vi "Execute Multiple Commands with a Single Channel with a Raspberry Pi.vi"() -> ()   [LabVIEW 2018]
doc: "Executes a multiple commands using a single channel with a Raspberry Pi as the remote SSH server. This is similar to connecting to a Raspberry Pi and executing multiple sequential commands. A more interactive experience, like a Read-Evaluate-Print-Loop (REPL), would require a while loop and some more complexity."
uses:
  Toolkit/Channel/Type Definitions/Terminals.ctl
  Toolkit/Channel/Channel.lvclass/Channel.ctl
  Toolkit/Session/Session.lvclass/Session.ctl
  Toolkit/SSH/SSH.lvclass/SSH.ctl
  Toolkit/Session/Utility/Read Shared Library.vi
  Toolkit/SSH/Utility/Read Shared Library.vi
  Toolkit/Session/Support/Create from SSH.vi
  Toolkit/Session/Support/Password Authentication.vi
  Toolkit/Channel/Support/Create from Session.vi
  Toolkit/Support/Check Status.vi
  Toolkit/Channel/Support/Destroy to Session.vi
  Toolkit/Session/Support/Destroy to SSH.vi
  Toolkit/SSH/SSH.lvclass
  Toolkit/Session/Session.lvclass
  Toolkit/Channel/Channel.lvclass
panel:
  out "Login Message":string
  out "Response 2":string
  in  "Command 2":string="echo \"Hello World from the second command!\""
  out "Response 1":string
  in  "Command 1":string="echo \"Hello World from the first command!\""
  in  "Raspberry Pi Address":string="raspberrypi.local"
  in  "Password":string
  in  "Username":string="pi"
  # "Overview: Demonstrates executing a multiple, sequential commands using a single Shell channel with a Raspberry Pi\nInstructions:\n1. Change the Raspberry Pi Address from the mDNS default to another mDNS or the IP address of the Raspberry Pi if needed.\n2. Change the username from the default Raspberry Pi user if needed.\n3. Enter the password for the Raspberry Pi user.\n4. Run this VI.\n5. Observe the login message from the Raspberry Pi.\n6. Observe \"Hello World from the first command!\" and \"Hello World from the second command!\" for Response 1 and 2, respectively.\n7. Change Command 1 and Command 2.\n8. Rerun this VI.\n9. Observe the responses for Command 1 and Command 2, respectively."
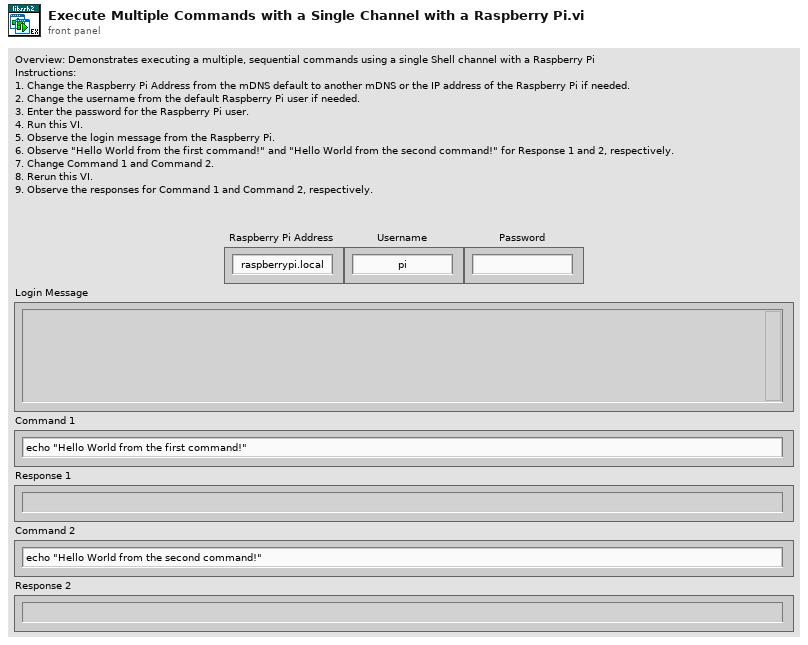
[diagram p1: front panel]
types:
  T1 = typedef "Toolkit.lvlib/Channel.lvclass/Terminals.ctl" = enum16{"ansi", "dump", "linux", "rxvt", "screen", "sun", "vt100", "vt102", "vt220", "vt52", "xterm"}
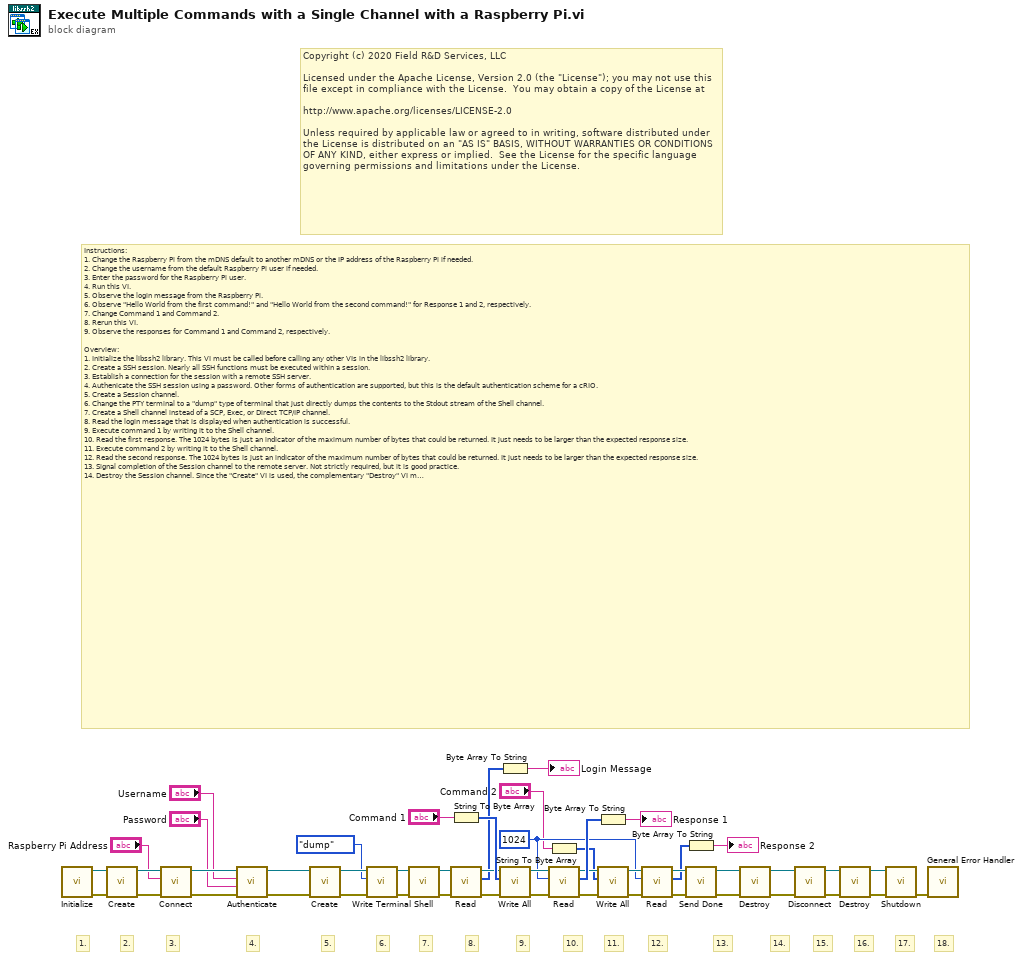
[diagram p0: block diagram]
diagram:
  w13 = u64 1024 ("Max Data Length")
  # "18."
  # "Copyright (c) 2020 Field R&D Services, LLC\n\nLicensed under the Apache License, Version 2.0 (the \"License\"); you may not use this file except in compliance with the License.  You may obtain a copy of the License at\n\nhttp://www.apache.org/licenses/LICENSE-2.0\n\nUnless required by applicable law or agreed to in writing, software distributed under the License is distributed on an \"AS IS\" BASIS, WITHOUT WARRANTIES OR CONDITIONS OF ANY KIND, either express or implied.  See the License for the specific language governing permissions and limitations under the License."
  # "17."
  # "16."
  # "15."
  # "14."
  # "13."
  # "12."
  # "11."
  # "10."
  # "9."
  # "8."
  # "7."
  # "6."
  # "5."
  # "4."
  # "3."
  # "2."
  # "1."
  # "Instructions:\n1. Change the Raspberry Pi from the mDNS default to another mDNS or the IP address of the Raspberry Pi if needed.\n2. Change the username from the default Raspberry Pi user if needed.\n3. Enter the password for the Raspberry Pi user.\n4. Run this VI.\n5. Observe the login message from the Raspberry Pi.\n6. Observe \"Hello World from the first command!\" and \"Hello World from the second command!\" for Response 1 and 2, respectively.\n7. Change Command 1 and Command 2.\n8. Rerun this VI.\n9. Observe the responses for Command 1 and Command 2, respectively.\n\nOverview:\n1. Initialize the libssh2 library. This VI must be called before calling any other VIs in the libssh2 library.\n2. Create a SSH session. Nearly all SSH functions must be executed within a session.\n3. Establish a connection for the session with a remote SSH server.\n4. Authenicate the SSH session using a password. Other forms of authentication are supported, but this is the default authentication scheme for a cRIO. \n5. Create a Session channel.\n6. Change the PTY terminal to a \"dump\" type of terminal that just directly dumps the contents to the Stdout stream of the Shell channel.\n7. Create a Shell channel instead of a SCP, Exec, or Direct TCP/IP channel.\n8. Read the login message that is displayed when authentication is successful.\n9. Execute command 1 by writing it to the Shell channel.\n10. Read the first response. The 1024 bytes is just an indicator of the maximum number of bytes that could be returned. It just needs to be larger than the expected response size.\n11. Execute command 2 by writing it to the Shell channel.\n12. Read the second response. The 1024 bytes is just an indicator of the maximum number of bytes that could be returned. It just needs to be larger than the expected response size.\n13. Signal completion of the Session channel to the remote server. Not strictly required, but it is good practice. \n14. Destroy the Session channel. Since the \"Create\" VI is used, the complementary \"Destroy\" VI must be used to free resources within the libssh2 library. \n15. Disconnect from the remote SSH server.\n16. Destroy the session to free resources within the libssh2 library.\n17. Shutdown the libssh2 library. This VI must be last VI called for the libssh2 library. No other libssh2 VIs should be called once this VI is executed.\n18. Provide some error handling and reporting. Libssh2 errors will be in the -8100 range."
  n1 = call "Initialize.vi"() -> ("Error Out"=w47:errorcluster, "SSH"=w48:refnum<class "SSH.lvclass">)  [unwired: 10 in]
  n2 = call-poly "Create.vi"("Error In"=w47, "SSH"=w48) -> ("Error Out"=w45:errorcluster, "Sesssion"=w46:refnum<class "Session.lvclass">)  [unwired: 8 in]
  n3 = call "Connect.vi"("Error In"=w45, "Address"="Raspberry Pi Address", "Session In"=w46) -> ("Error Out"=w43:errorcluster, "Sesssion Out"=w44:refnum<class "Session.lvclass">)  [unwired: 7 in]
  n4 = call-poly "Authenticate.vi"("Error In"=w43, "Password"="Password", "Username"="Username", "Session In"=w44) -> ("Error Out"=w41:errorcluster, "Sesssion Out"=w42:refnum<class "Session.lvclass">)  [unwired: 6 in]
  n5 = call-poly "Create.vi"("Error In"=w41, "Session"=w42) -> ("Error Out"=w24:errorcluster, "Channel"=w25:refnum<class "Channel.lvclass">)  [unwired: 8 in]
  n6 = call "Write Terminal.vi"("Error In"=w24, "Terminal"=Terminals."dump", "Channel In"=w25) -> ("Error Out"=w8:errorcluster, "Channel Out"=w9:refnum<class "Channel.lvclass">)  [unwired: 7 in]
  n7 = call "Shell.vi"("Error In"=w8, "Channel In"=w9) -> ("Error Out"=w5:errorcluster, "Channel Out"=w3:refnum<class "Channel.lvclass">)  [unwired: 8 in]
  n8 = String To Byte Array(string="Command 1") -> (unsigned byte array=w22:u8[])
  n9 = call "Read.vi"("Error In"=w5, "Channel In"=w3) -> ("Error Out"=w4:errorcluster, "Data"=w1:u8[], "Channel Out"=w6:refnum<class "Channel.lvclass">)  [unwired: 7 in]
  n10 = Byte Array To String(unsigned byte array=w1) -> (string=→"Login Message":string)
  n11 = call "Write All.vi"("Error In"=w4, "Data"=w22, "Channel In"=w6) -> ("Error Out"=w20:errorcluster, "Channel Out"=w21:refnum<class "Channel.lvclass">)  [unwired: 6 in, 1 out]
  n12 = String To Byte Array(string="Command 2") -> (unsigned byte array=w10:u8[])
  n13 = call "Read.vi"("Error In"=w20, "Max Data Length"=w13, "Channel In"=w21) -> ("Error Out"=w18:errorcluster, "Data"=w32:u8[], "Channel Out"=w19:refnum<class "Channel.lvclass">)  [unwired: 6 in]
  n14 = Byte Array To String(unsigned byte array=w32) -> (string=→"Response 1":string)
  n15 = call "Write All.vi"("Error In"=w18, "Data"=w10, "Channel In"=w19) -> ("Error Out"=w16:errorcluster, "Channel Out"=w17:refnum<class "Channel.lvclass">)  [unwired: 6 in, 1 out]
  n16 = call "Read.vi"("Error In"=w16, "Max Data Length"=w13, "Channel In"=w17) -> ("Error Out"=w15:errorcluster, "Data"=w12:u8[], "Channel Out"=w14:refnum<class "Channel.lvclass">)  [unwired: 6 in]
  n17 = Byte Array To String(unsigned byte array=w12) -> (string=→"Response 2":string)
  n18 = call "Send Done.vi"("Error In"=w15, "Channel In"=w14) -> ("Error Out"=w39:errorcluster, "Channel Out"=w40:refnum<class "Channel.lvclass">)  [unwired: 8 in]
  n19 = call-poly "Destroy.vi"("Error In"=w39, "Channel"=w40) -> ("Error Out"=w37:errorcluster, "Session"=w38:refnum<class "Session.lvclass">)  [unwired: 8 in]
  n20 = call "Disconnect.vi"("Error In"=w37, "Session In"=w38) -> ("Error Out"=w35:errorcluster, "Sesssion Out"=w36:refnum<class "Session.lvclass">)  [unwired: 8 in]
  n21 = call-poly "Destroy.vi"("Error In"=w35, "Session"=w36) -> ("Error Out"=w33:errorcluster, "SSH"=w34:refnum<class "SSH.lvclass">)  [unwired: 8 in]
  n22 = call "Shutdown.vi"("Error In"=w33, "SSH"=w34) -> ("Error Out"=w27:errorcluster)  [unwired: 9 in]
  n23 = call <vilib>:"General Error Handler.vi"("error in (no error)"=w27) -> ()  [unwired: 10 in, 5 out]
